vi "VisualizedPoints.vi"(10 "WaypointsOverride":cluster{"x":dbl, "y":dbl, "th":dbl}[](array[cluster])) -> (2 "WaypointsOverride 2":cluster{"x":dbl, "y":dbl, "th":dbl}[](array[cluster]))   [LabVIEW 2025]
doc: "This VI starts when test mode begins, and will automatically be terminated when it ends. It will automatically publish I/O values, and you can add manual tests that can be invoked from the dashboard."
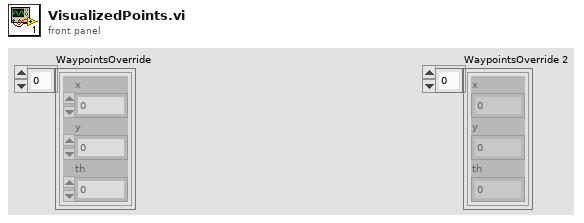
[diagram p1: front panel]
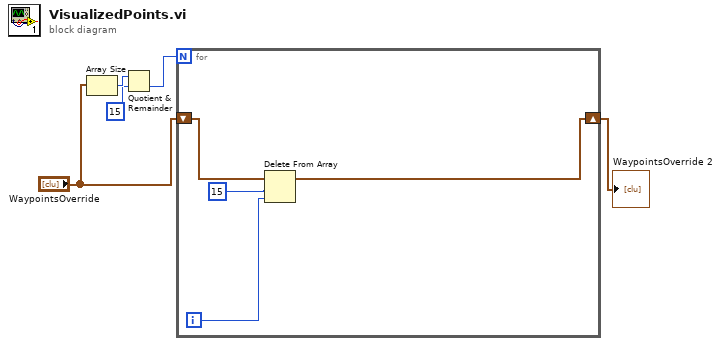
[diagram p0: block diagram]
diagram:
  n1 = Array Size(array="WaypointsOverride") -> (size(s)=w3:i32)
  n2 = Quotient & Remainder(x=w3, y=15) -> (floor(x/y)=w1:i32)  [unwired: 1 out]
  n3 = for {
    N: w1 -> [_]
    shift-right: [w6] -> w5
    shift-left: "WaypointsOverride" -> [w9]
    i -> [w7]
    n4 = Delete From Array(array=w9, length=15, index=w7) -> (array with subset deleted=w6:cluster{"x":dbl, "y":dbl, "th":dbl}[])  [unwired: 1 out]
  }
  "WaypointsOverride 2" <- w5
